vi "(TestVI)Accelerometer Test.vi"() -> ()   [LabVIEW 2020]
uses:
  SubVIs/Serial/Controls/(Ctrl)Serial_FGV Function.ctl
  <vilib>/Instr/_visa.llb/VISA Find Search Mode.ctl
  SubVIs/I2C/Instance VIs/(SubVI)I2C_8Bit-8Bit_Read_Sequential.vi
  SubVIs/I2C/Instance VIs/(SubVI)I2C_8Bit-8Bit_Read_Single.vi
  SubVIs/I2C/Instance VIs/(SubVI)I2C_8Bit-8Bit_Write_Single.vi
panel:
  out "FIFO Entries":u8
  in  "Read":bool
  in  "Start Address 2":u8 format="%02x"
  out "Data to Write 2":u8 format="%02x"
  out "*(타입 *) &x 2":i16[](array[numeric]) format="%d\n0x%04x"
  in  "Read Acc":bool
  in  "Data to Write":u8 format="%02x"
  in  "Start Address":u8 format="%02x"
  in  "Write":bool
  in  "정지":bool
  out "*(타입 *) &x":u8[](array[numeric]) format="%.0x"
  in  "Read All":bool
  in  "ID":u8=166 format="%02x"
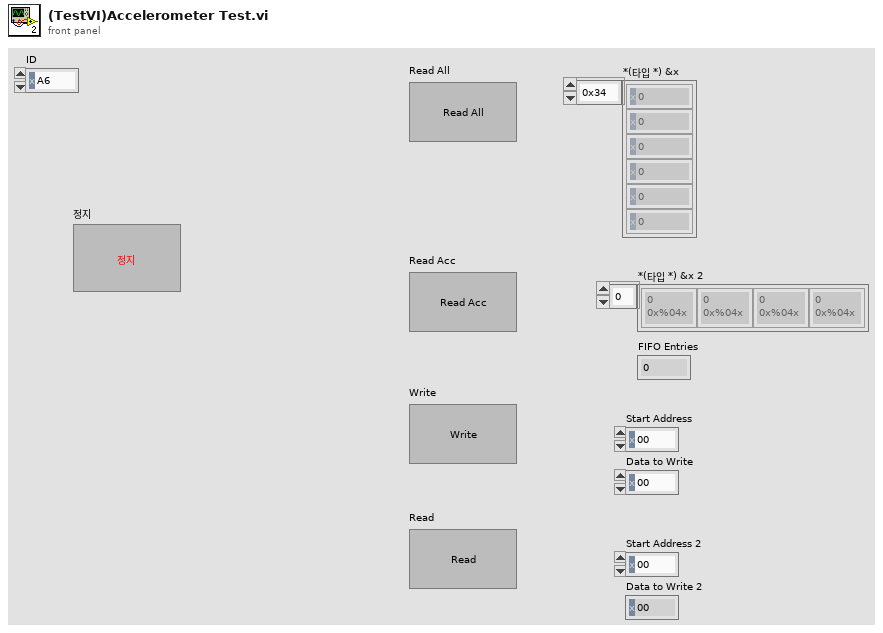
[diagram p1: front panel]
types:
  T1 = typedef "VISA Find Search Mode.ctl" = u32
  T2 = typedef "(Ctrl)Serial_FGV Function.ctl" = enum16{"Initialize", "Read", "Read All", "Write", "Flush Buffer", "Get Ref.", "Close"}
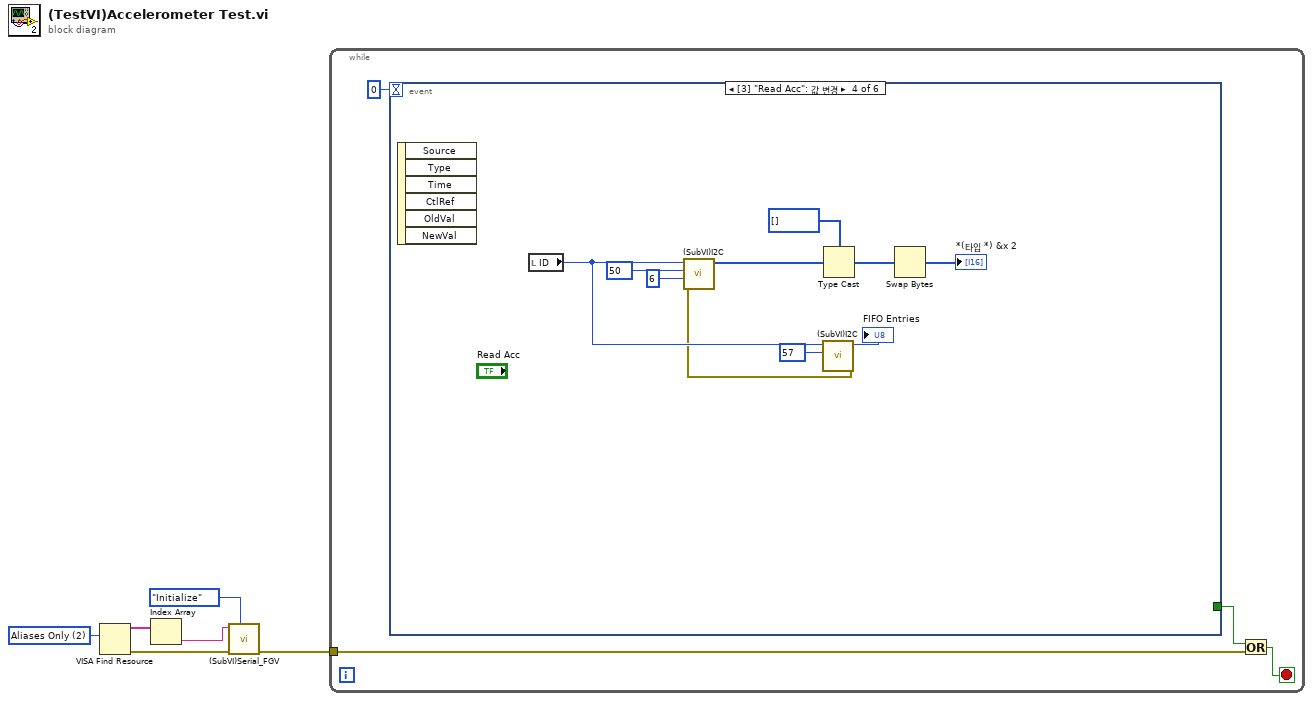
[diagram p0: block diagram]
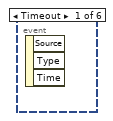
[diagram p2: hidden frame]
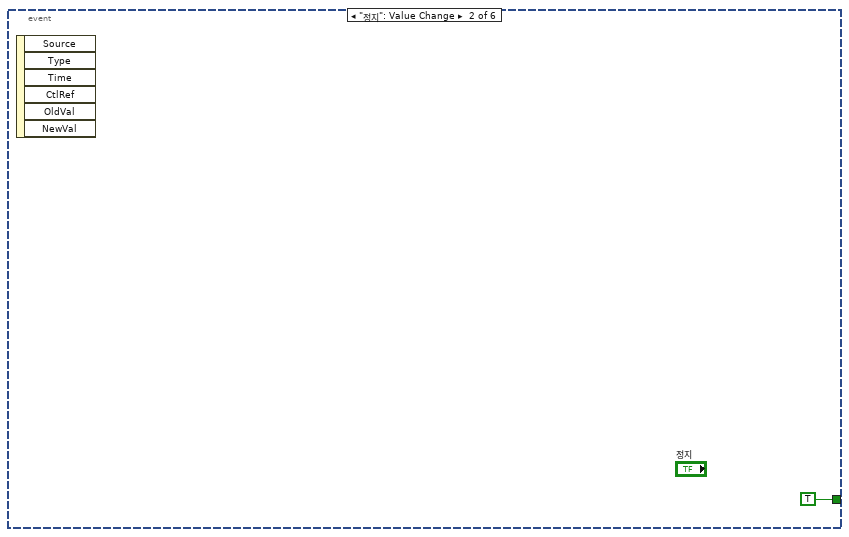
[diagram p3: hidden frame]
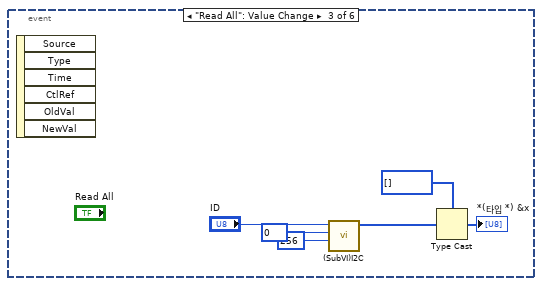
[diagram p4: hidden frame]
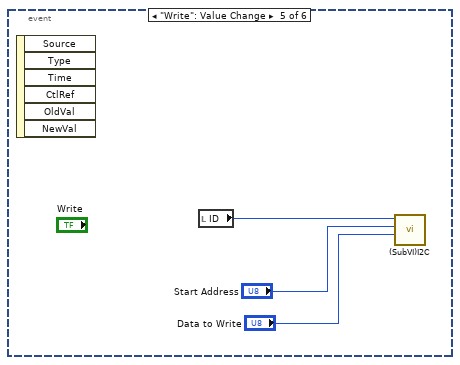
[diagram p5: hidden frame]
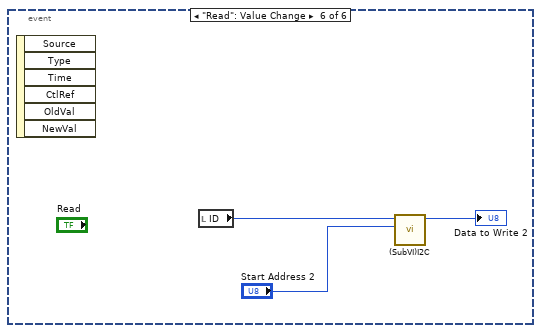
[diagram p6: hidden frame]
diagram:
  w5 = T1 2 items=["Canonical Names Only"=0, "Aliases Only"=2, "Include Matching Aliases"=3, "Include All Aliases"=4] ("Search Mode")
  n1 = VISA Find Resource(10:w5) -> (0:w4:errorcluster, 3:w3:string[])  [unwired: 2 in, 1 out]
  n2 = Index Array(array=w3) -> (element=w2:string)  [unwired: 1 in]
  n3 = call "(SubVI)Serial_FGV.vi"("Function"=(Ctrl)Serial_FGV_Function."Initialize", "error in (no error)"=w4, "VISA resource name"=w2) -> ("error out"=w1:errorcluster)  [unwired: 6 in, 2 out]
  n4 = while {
    tunnel: w1 -> [w9]
    stop <- w8 stop-if-true
    n5 = event shown="[3] \"Read Acc\": 값 변경" {
      selector: _ -> [_ _ _ _ _ _]
      dyn-events: _ -> [_ _ _ _ _ _]
      timeout: 0 -> [_ _ _ _ _ _]
      tunnel: [_ TRUE _ _ _ _] -> w7
      event Timeout {
        n6 = event-data() -> ()  [unwired: 1 in, 3 out]
      }
      event "정지": Value Change {
        n7 = event-data() -> ()  [unwired: 1 in, 6 out]
      }
      event "Read All": Value Change {
        n8 = event-data() -> ()  [unwired: 1 in, 6 out]
        n9 = call-poly "(SubVI)I2C.vi"("Size to Read"=u16 256, "Start Address"=u8 0, "ID"="ID") -> ("Read Data"=w14:u8[])  [unwired: 6 in, 2 out]
        n10 = Type Cast(type=u8[] [] ("타입"), x=w14) -> (*(type *) &x=→"*(타입 *) &x":u8[])
      }
      event "Read Acc": Value Change {
        n11 = event-data() -> ()  [unwired: 1 in, 6 out]
        n12 = local read "ID"() -> (w21:u8)
        n13 = call-poly "(SubVI)I2C.vi"("Address"=u8 57 ("Start Address"), "ID"=w21) -> ("error out"=w18:errorcluster, "Read Data"=→"FIFO Entries":u8)  [unwired: 7 in, 1 out]
        n14 = call-poly "(SubVI)I2C.vi"("error in (no error)"=w18, "Size to Read"=u16 6, "Start Address"=u8 50, "ID"=w21) -> ("Read Data"=w27:u8[])  [unwired: 5 in, 2 out]
        n15 = Type Cast(type=i16[] [] ("타입"), x=w27) -> (*(type *) &x=w26:i16[])
        n16 = Swap Bytes(anything=w26) -> (byte swapped=→"*(타입 *) &x 2":i16[])
      }
      event "Write": Value Change {
        n17 = event-data() -> ()  [unwired: 1 in, 6 out]
        n18 = local read "ID"() -> (w29:u8)
        n19 = call-poly "(SubVI)I2C.vi"("Data to Write"="Data to Write", "Address"="Start Address", "ID"=w29) -> ()  [unwired: 7 in, 2 out]
      }
      event "Read": Value Change {
        n20 = event-data() -> ()  [unwired: 1 in, 6 out]
        n21 = local read "ID"() -> (w32:u8)
        n22 = call-poly "(SubVI)I2C.vi"("Address"="Start Address 2", "ID"=w32) -> ("Read Data"=→"Data to Write 2":u8)  [unwired: 7 in, 2 out]
      }
    }
    n23 = Or(x=w7, y=w9) -> (x .or. y?=w8:bool)
  }
